vi "test stop.vi"() -> ()   [LabVIEW 2019]
panel:
  out "error out 4":errorcluster
  in  "OK Button":bool
  in  "String":string
  out "Application:All VIs In Memory":string[](array[string])
  out "error out 3":errorcluster
  out "Front Panel Window:State":T1(ring)
  out "error out 2":errorcluster
  out "error out":errorcluster
  in  "Open":bool
  in  "Stop":bool
  in  "Abort":bool
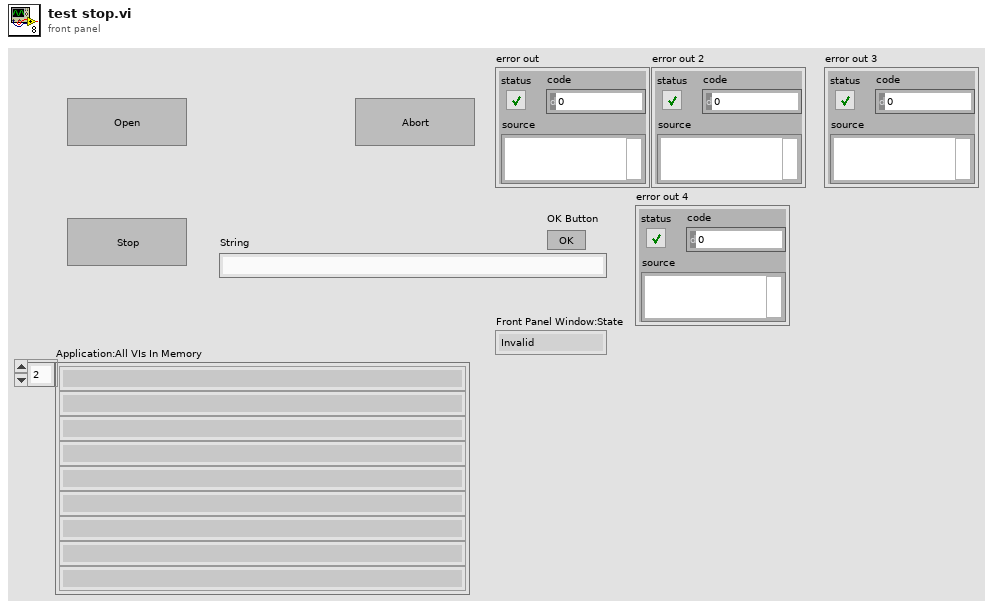
[diagram p1: front panel]
types:
  T1 = enum32{"Invalid", "Standard", "Closed", "Hidden", "Minimized", "Maximized"}
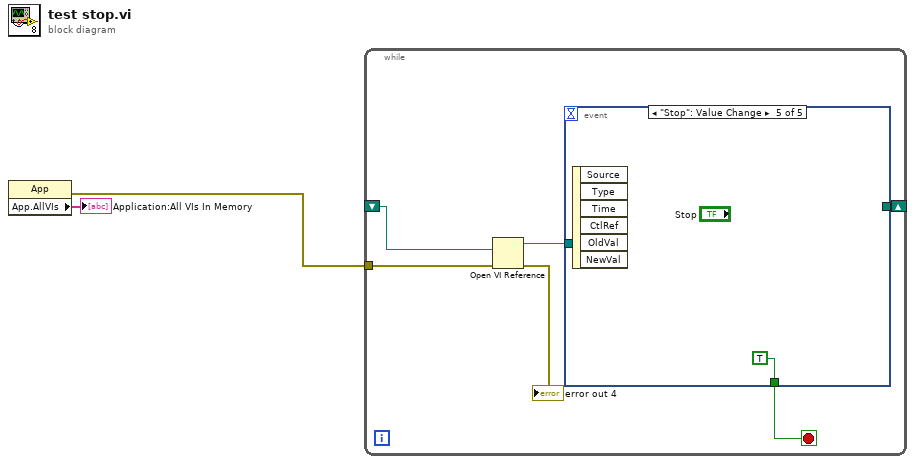
[diagram p0: block diagram]
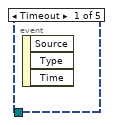
[diagram p2: hidden frame]
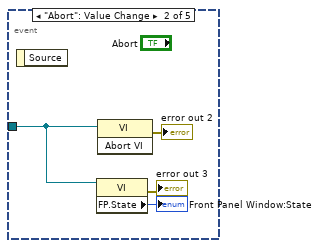
[diagram p3: hidden frame]
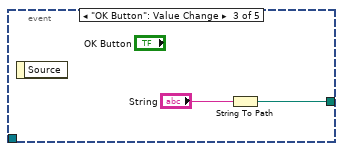
[diagram p4: hidden frame]
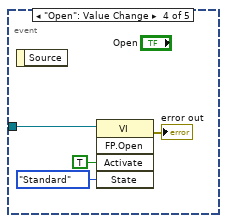
[diagram p5: hidden frame]
diagram:
  n1 = property class="App"() -> (error out=w1:errorcluster, "App.AllVIs"=→"Application:All VIs In Memory":string[])  [unwired: 2 in, 1 out]
  n2 = while {
    shift-right: [w6] -> _
    shift-left: _ -> [w5]
    tunnel: w1 -> [w3]
    stop <- w8 stop-if-true
    n3 = Open VI Reference(vi path=w5, error in (no error)=w3) -> (vi reference=w7:refnum<vi>, error out=→"error out 4":errorcluster)  [unwired: 4 in]
    n4 = event shown="[4] \"Stop\": Value Change" {
      selector: _ -> [_ _ _ _ _]
      dyn-events: _ -> [_ _ _ _ _]
      timeout: _ -> [_ _ _ _ _]
      tunnel: w7 -> [_ w11 _ w18 _]
      tunnel: [_ _ _ _ TRUE] -> w8
      tunnel: [_ _ w13 _ _] -> w6
      event Timeout {
        n5 = event-data() -> ()  [unwired: 1 in, 3 out]
      }
      event "Abort": Value Change {
        n6 = event-data() -> ()  [unwired: 1 in, 1 out]
        n7 = property class="VI"(reference=w11) -> (error out=→"error out 3":errorcluster, "FP.State"=→"Front Panel Window:State":T1)  [unwired: 1 in, 1 out]
        n8 = invoke class="VI" method="Abort VI"(reference=w11) -> (error out=→"error out 2":errorcluster)  [unwired: 2 in, 2 out]
      }
      event "OK Button": Value Change {
        n9 = event-data() -> ()  [unwired: 1 in, 1 out]
        n10 = String To Path(string="String") -> (path=w13:path)
      }
      event "Open": Value Change {
        n11 = event-data() -> ()  [unwired: 1 in, 1 out]
        n12 = invoke class="VI" method="FP.Open"(reference=w18, "Activate"=TRUE ("Activate?"), "State"=T1."Standard") -> (error out=→"error out":errorcluster)  [unwired: 2 in, 4 out]
      }
      event "Stop": Value Change {
        n13 = event-data() -> ()  [unwired: 1 in, 6 out]
      }
    }
  }
